vi "WPI_RobotDriveOpen6MotorWithCANJaguar.vi"(0 "Rear Left Motor":u8, 1 "Rear Right Motor":u8, 2 "Front Right Motor":u8, 3 "Front Left Motor":u8, 4 "Mid Left Motor":u8, 5 "error in (no error)":errorcluster, 6 "Mid Right Motor":u8, 9 "Left Motors Inverted":bool, 11 "Right Motors Inverted":bool) -> (14 "RobotDriveDevRef":T1={"DevStatus"={"status"=FALSE, "code"=0, "source"=""}, "Motors[]"=[], "Square Inputs"=FALSE, "Max Output"=1.0, "Isochronous"=FALSE}, 19 "error out":errorcluster)   [LabVIEW 2013]
doc: "Opens a reference to the robot drive for a four-motor robot using CAN Jaguar motor controllers.\n\nThe CAN Jaguars are opened in Percent VBus mode. \n\nThis software is licensed. Open the labview\\readme\\WPI Robotics Library Open Source License.txt file for more information."
uses:
  <vilib>/Rock Robotics/WPI/RobotDrive/WPI_RobotDriveDevRef.ctl
  <vilib>/Rock Robotics/WPI/MotorControl/WPI_MotorControlDeviceRef.ctl
  <vilib>/Rock Robotics/SystemInterfaces/Typedef/FPGA_TypedefDigitalModule.ctl
  <vilib>/Rock Robotics/SystemInterfaces/DIO/FPGA_DIOPWMChannel.ctl
  <vilib>/Rock Robotics/WPI/PWM/WPI_PWMDeadband.ctl
  <vilib>/Rock Robotics/WPI/CAN/Jaguar/SubVIs/WPI_CANJaguar_ControlMode.ctl
  <vilib>/Rock Robotics/WPI/PWM/WPI_PWMTransform_ConPane.ctl
  <vilib>/Rock Robotics/WPI/SafetyOutput/WPI_SafetyOutputConfigMenu.ctl
  <vilib>/Rock Robotics/WPI/MotorControl/WPI_MotorControlOpenCANJaguar.vi
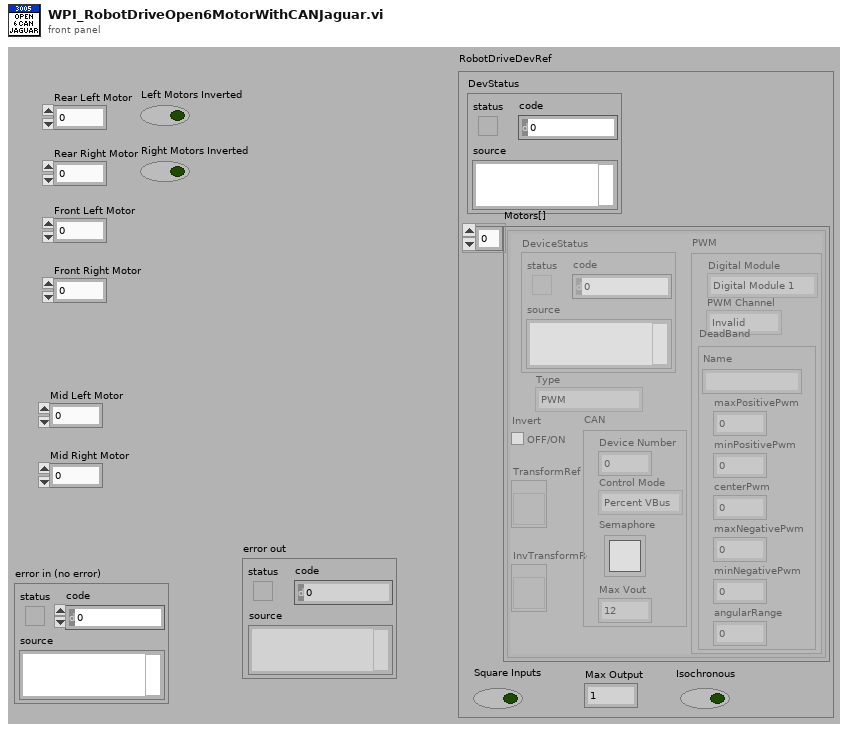
[diagram p1: front panel]
types:
  T1 = typedef "WPI_RobotDriveDevRef.ctl" = cluster{"DevStatus":errorcluster, "Motors[]":T2[], "Square Inputs":bool, "Max Output":dbl, "Isochronous":bool}
  T2 = typedef "WPI_MotorControlDeviceRef.ctl" = cluster{"DeviceStatus":errorcluster, "Type":enum16{"PWM", "CAN"}, "PWM":cluster{"Digital Module":T3, "PWM Channel":T4, "DeadBand":T5}, "CAN":cluster{"Device Number":u8, "Control Mode":T6, "Semaphore":T7, "Max Vout":dbl}, "Invert":bool, "TransformRef":T8, "InvTransformRef":T8}
  T3 = typedef "FPGA_TypedefDigitalModule.ctl" = enum16{"Digital Module 1", "Digital Module 2"}
  T4 = typedef "FPGA_DIOPWMChannel.ctl" = enum8{"PWM 1", "PWM 2", "PWM 3", "PWM 4", "PWM 5", "PWM 6", "PWM 7", "PWM 8", "PWM 9", "PWM 10", "Invalid"}
  T5 = typedef "WPI_PWMDeadband.ctl" = cluster{"Name":string, "maxPositivePwm":i32, "minPositivePwm":i32, "centerPwm":i32, "maxNegativePwm":i32, "minNegativePwm":i32, "angularRange":u16}
  T6 = typedef "WPI_CANJaguar_ControlMode.ctl" = enum8{"Percent VBus", "Current", "Speed", "Position", "Voltage"}
  T7 = typedef "Semaphore RefNum" = refnum<k1>
  T8 = typedef "WPI_PWMTransform_ConPane.ctl" = refnum<vi>
  T9 = typedef "WPI_SafetyOutputConfigMenu.ctl" = enum16{"Enable", "Disable"}
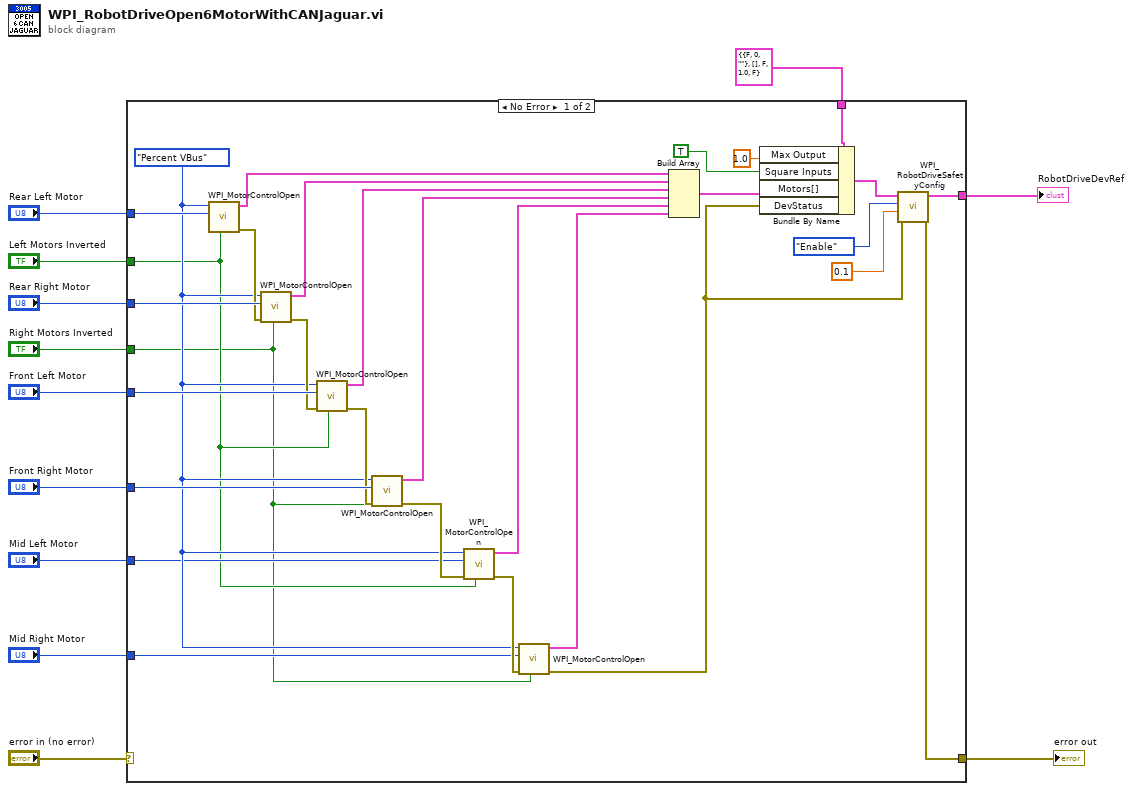
[diagram p0: block diagram]
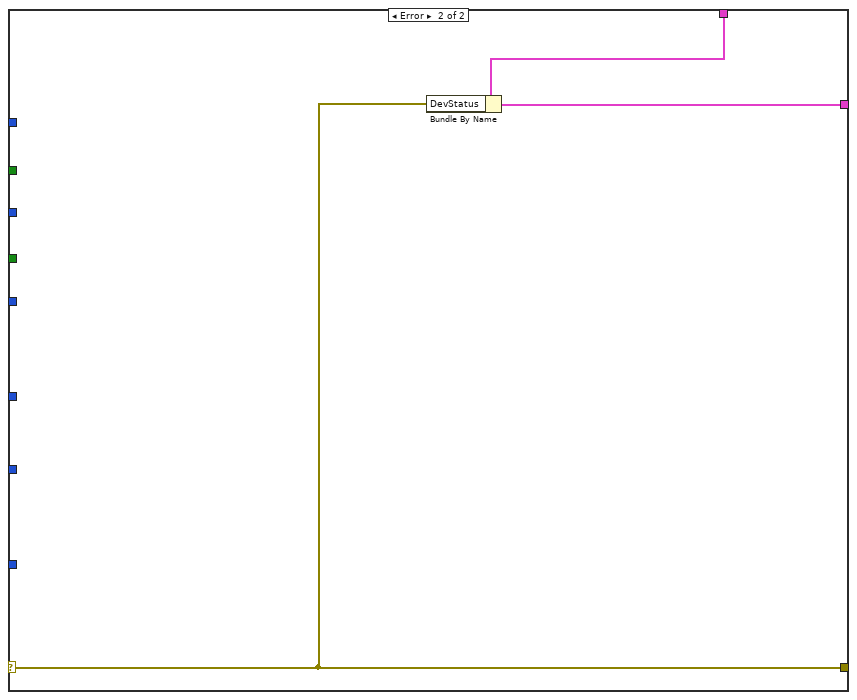
[diagram p2: hidden frame]
diagram:
  n1 = case shown="No Error" "error in (no error)" {
    selector: "error in (no error)" -> [_ w43]
    tunnel: [w25 w44] -> w12
    tunnel: T1 {"DevStatus"={"status"=FALSE, "code"=0, "source"=""}, "Motors[]"=[], "Square Inputs"=FALSE, "Max Output"=1.0, "Isochronous"=FALSE} ("RobotDriveDevRef") -> [w42 w45]
    tunnel: "Rear Left Motor" -> [w40 _]
    tunnel: "Front Right Motor" -> [w37 _]
    tunnel: "Front Left Motor" -> [w38 _]
    tunnel: "Rear Right Motor" -> [w39 _]
    tunnel: "Left Motors Inverted" -> [w14 _]
    tunnel: "Right Motors Inverted" -> [w13 _]
    tunnel: [w26 w43] -> w3
    tunnel: "Mid Left Motor" -> [w16 _]
    tunnel: "Mid Right Motor" -> [w15 _]
    frame No Error {
      w17 = WPI_CANJaguar_ControlMode."Percent VBus" ("Control Mode")
      n2 = call-poly <vilib>:"WPI_MotorControlOpen.vi"("Invert"=w14, "Device Number"=w40, "Control Mode"=w17) -> ("error out"=w30:errorcluster, "MotorControlDeviceRef"=w36:T2)  [unwired: 3 in, 4 out]
      n3 = call-poly <vilib>:"WPI_MotorControlOpen.vi"("Invert"=w13, "error in (no error)"=w30, "Device Number"=w39, "Control Mode"=w17) -> ("error out"=w31:errorcluster, "MotorControlDeviceRef"=w35:T2)  [unwired: 2 in, 4 out]
      n4 = call-poly <vilib>:"WPI_MotorControlOpen.vi"("Invert"=w14, "error in (no error)"=w31, "Device Number"=w38, "Control Mode"=w17) -> ("error out"=w32:errorcluster, "MotorControlDeviceRef"=w34:T2)  [unwired: 2 in, 4 out]
      n5 = call-poly <vilib>:"WPI_MotorControlOpen.vi"("Invert"=w13, "error in (no error)"=w32, "Device Number"=w37, "Control Mode"=w17) -> ("error out"=w21:errorcluster, "MotorControlDeviceRef"=w33:T2)  [unwired: 2 in, 4 out]
      n6 = call-poly <vilib>:"WPI_MotorControlOpen.vi"("Invert"=w14, "error in (no error)"=w21, "Device Number"=w16, "Control Mode"=w17) -> ("error out"=w22:errorcluster, "MotorControlDeviceRef"=w20:T2)  [unwired: 2 in, 4 out]
      n7 = call-poly <vilib>:"WPI_MotorControlOpen.vi"("Invert"=w13, "error in (no error)"=w22, "Device Number"=w15, "Control Mode"=w17) -> ("error out"=w18:errorcluster, "MotorControlDeviceRef"=w19:T2)  [unwired: 2 in, 4 out]
      n8 = Build Array(w36, w35, w34, w33, w20, w19) -> (w29:T2[])
      n9 = Bundle By Name(cluster=w42, "Max Output"=1.0, "Square Inputs"=TRUE ("DestroyPWM?"), "Motors[]"=w29, "DevStatus"=w18) -> (w27:T1)
      n10 = call <vilib>:"WPI_RobotDriveSafetyConfig.vi"("error in (no error)"=w18, "timeout (s)"=0.1, "mode"=WPI_SafetyOutputConfigMenu."Enable", "RobotDriveDevRef"=w27) -> ("error out"=w26:errorcluster, "RobotDriveDevRef"=w25:T1)  [unwired: 6 out]
    }
    frame Error {
      n11 = Bundle By Name(cluster=w45, "DevStatus"=w43) -> (w44:T1)
    }
  }
  "RobotDriveDevRef" <- w12
  "error out" <- w3
